vi "CRYReport Part ObjectDblClicked Event Callback.vi"(4 "TXTextControl":refnum<k7>, 5 "Event Data":cluster{"ObjectId":i16}, 6 "Control Ref":refnum<k7>, 7 "Event Common Data":T1) -> ()   [LabVIEW 2013]
uses:
  CRYReport Global.vi
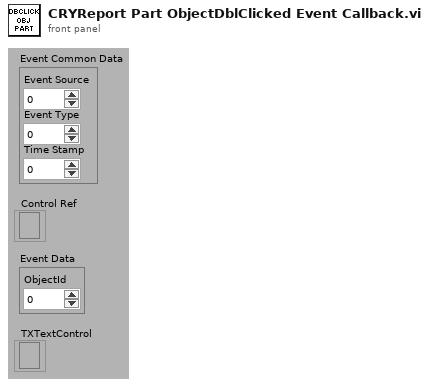
[diagram p1: front panel]
types:
  T1 = cluster{"Event Source":i32, "Event Type":u32, "Time Stamp":u32}
  T2 = cluster{"nID":i16, "sName":string, "pVIRef":refnum<vi>, "pSPRef":refnum<vi>, "sTitle":string, "nIDObject":i16, "nIDV":i16, "nWidth":i16, "nHeight":i16, "bImgChange":bool, "sType":string, "sState":string, "sPosition":string, "sData":string}
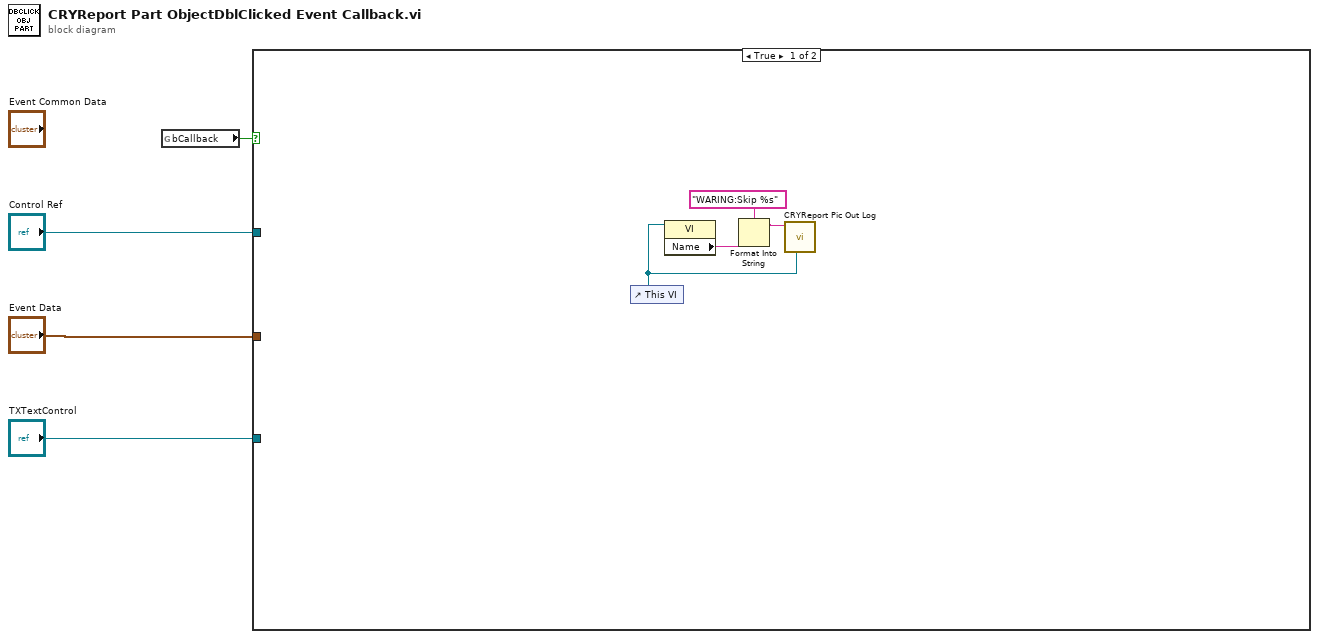
[diagram p0: block diagram]
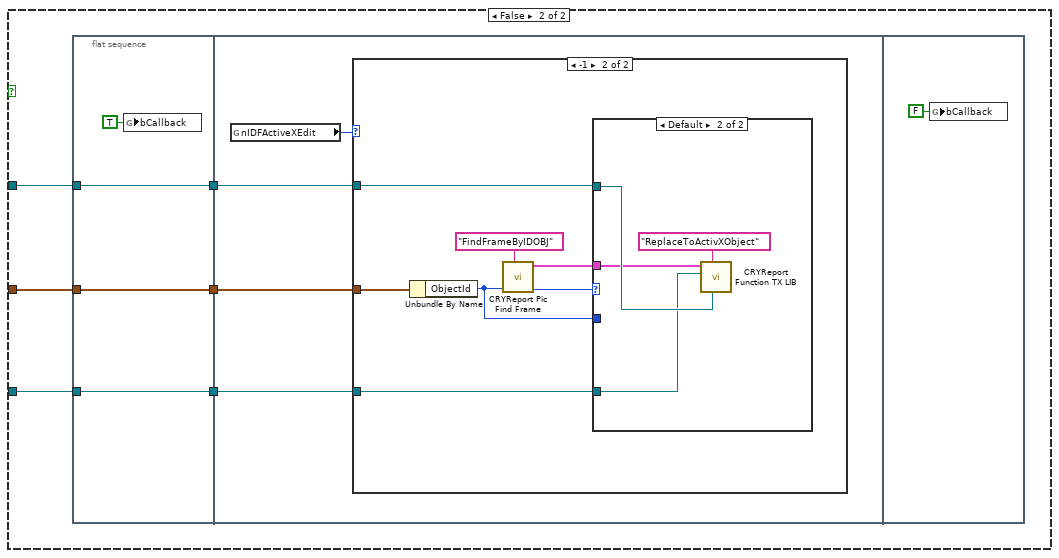
[diagram p2: hidden frame]
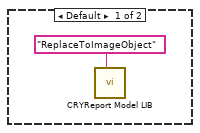
[diagram p3: hidden frame]
diagram:
  n1 = global read "CRYReport Global.vi" "bCallback"() -> (w1:bool)
  n2 = case shown="True" w1 {
    tunnel: "Event Data" -> [_ w14]
    tunnel: "Control Ref" -> [_ w13]
    tunnel: "TXTextControl" -> [_ w12]
    frame True {
      n3 = control-ref of="This VI"() -> (w5:refnum<vi>)
      n4 = property class="VI"(reference=w5) -> ("Name"=w6:string)  [unwired: 1 in, 2 out]
      n5 = Format Into String(format string="WARING:Skip %s" ("string"), w6) -> (resulting string=w8:string)  [unwired: 2 in, 1 out]
      n6 = call "CRYReport Pic Out Log.vi"("vi reference"=w5, "sData"=w8) -> ()  [unwired: 10 in]
    }
    frame False {
      n7 = flat-sequence {
        tunnel: w12 -> [w16]
        tunnel: w13 -> [w17]
        tunnel: w14 -> [w18]
        tunnel: [w18] -> w11
        tunnel: [w17] -> w10
        tunnel: [w16] -> w9
        tunnel: w11 -> [w22]
        tunnel: w10 -> [w21]
        tunnel: w9 -> [w20]
        frame #0 {
          n8 = global write "CRYReport Global.vi" "bCallback"(TRUE ("bCallback")) -> ()
        }
        frame #1 {
          n9 = global read "CRYReport Global.vi" "nIDFActiveXEdit"() -> (w19:i16)
          n10 = case shown="-1" w19 {
            tunnel: w22 -> [_ w27]
            tunnel: w21 -> [_ w26]
            tunnel: w20 -> [_ w25]
            frame Default {
              n11 = call "CRYReport Model LIB.vi"("sAction"="ReplaceToImageObject") -> ()  [unwired: 9 in, 2 out]
            }
            frame -1 {
              n12 = Unbundle By Name(w27) -> ("ObjectId"=w24:i16)
              n13 = call "CRYReport Pic Find Frame.vi"("sAction"="FindFrameByIDOBJ", "nData"=w24) -> ("nData_Out"=w28:i32, "cFrame_Out"=w29:T2)  [unwired: 8 in]
              n14 = case shown="Default" w28 {
                tunnel: w29 -> [_ w31]
                tunnel: w26 -> [_ w33]
                tunnel: w25 -> [_ w32]
                tunnel: w24 -> [_ _]
                frame -1 {
                }
                frame Default {
                  n15 = call "CRYReport Function TX LIB.vi"("Control Ref"=w33, "sAction"="ReplaceToActivXObject", "TXTextControl"=w32, "cFrame"=w31) -> ()  [unwired: 5 in, 3 out]
                }
              }
            }
          }
        }
        frame #2 {
          n16 = global write "CRYReport Global.vi" "bCallback"(FALSE ("bCallback")) -> ()
        }
      }
    }
  }
